vi "CDF Mechanism Controller.vi"(8 "error in":errorcluster) -> ()   [LabVIEW 2015]
doc: "This VI executes continuously carrying out the current operation and responding to updates or new operations. It will often contain the timing or control code that is difficult to place directly in TeleOp. This VI generally opens all sensors and motors and isolates the rest of the robot code from knowing how the operations are carried out."
uses:
  CDF Mechanism Setpoints.ctl
  CDF Mechanism Operations.ctl
  <vilib>/Rock Robotics/WPI/CAN/TalonSRX/WPI_CANTalonSRX_APIControlMode.ctl
  <vilib>/Rock Robotics/WPI/CAN/TalonSRX/WPI_CANTalonSRX_BrakeOverride.ctl
  <vilib>/Rock Robotics/WPI/CAN/TalonSRX/WPI_CANTalonSRX_APIFeedbackSelect.ctl
  Support Code/OnButton/OnButtonSingle.vi
  <vilib>/Rock Robotics/WPI/MotorControl/WPI_MotorControlOpenCANTalonSRX.vi
panel:
  out "Current\nCmd":string
  # "Tip: It may be helpful to observe inputs and sensor values.\nYou may also want to display tuning or debugging controls."
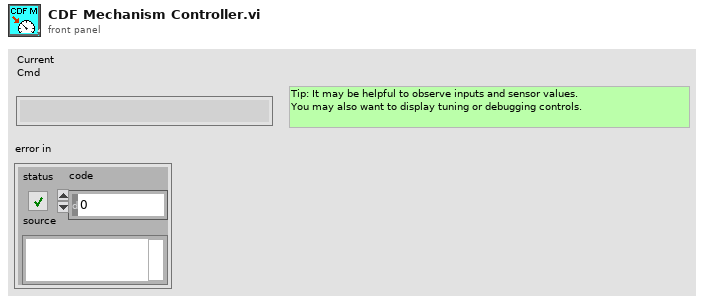
[diagram p1: front panel]
types:
  T1 = typedef "CDF Mechanism Setpoints.ctl" = cluster{"Operation":T2, "Setpoint":dbl, "Duration":dbl, "Setpoint (Top is = True )":bool}
  T2 = typedef "CDF Mechanism Operations.ctl" = enum16{"Reserve", "Read Current", "Immediate", "Idle", "Flip", "Set", "Manual"}
  T3 = typedef "Command Status Info.ctl" = cluster{"Name":string, "Status":T4, "notifier out":T5}
  T4 = typedef "Completion Status.ctl" = enum16{"Successful", "Aborted", "Incomplete"}
  T5 = typedef "Completion Notifier.ctl" = refnum<notifier>
  T6 = cluster{"Default Command":T1, "Command Timing":cluster{"Start Time (ms)":u32, "Iterations":i32}, "Command Arguments":cluster{"Command Info":T3, "Description":string, "Default Command":T1, "notifier out":refnum<notifier>, "Subsystem Name":string}}
  T7 = typedef "WPI_CANTalonSRX_APIFeedbackSelect.ctl" = enum16{"Digital Quadrature Encoder", "Analog Potentiometer", "Analog Encoder", "Count on Quad-A (Rising-Edge)", "Count on Quad-A (Falling-Edge)", "CTR Magnetic Enc (Absolute)", "CTR Magnetic Enc (Relative)", "Pulse Width"}
  T8 = typedef "WPI_CANTalonSRX_BrakeOverride.ctl" = enum8{"No Override", "Override to Coast", "Override to Brake"}
  T9 = typedef "WPI_CANTalonSRX_APIControlMode.ctl" = enum8{"Percent VBus", "Speed", "Position", "Slave", "Unchanged / Invalid", "Voltage Compensation", "Current", "Motion Profile"}
  T10 = typedef "WPI_MotorControlDeviceRef.ctl" = cluster{"DeviceStatus":errorcluster, "Type":T11, "PWM":cluster{"PWM Channel":T12, "DeadBand":T13}, "CAN":cluster{"Device Number":u8, "Control Mode":T14, "Semaphore":T15, "Max Vout":dbl, "TalonSRX Control Mode":T9}, "Invert":bool}
  T11 = typedef "WPI_MotorControlType.ctl" = enum16{"PWM", "CAN", "CANTalonSRX"}
  T12 = typedef "FPGA_DIOPWMChannel.ctl" = enum8{"PWM 0", "PWM 1", "PWM 2", "PWM 3", "PWM 4", "PWM 5", "PWM 6", "PWM 7", "PWM 8", "PWM 9", "PWM MXP 0", "PWM MXP 1", "PWM MXP 2", "PWM MXP 3", "PWM MXP 4", "PWM MXP 5", "PWM MXP 6", "PWM MXP 7", "PWM MXP 8", "PWM MXP 9", "Invalid"}
  T13 = typedef "WPI_PWMDeadband.ctl" = cluster{"Name":string, "maxPositivePwm":i32, "minPositivePwm":i32, "centerPwm":i32, "maxNegativePwm":i32, "minNegativePwm":i32, "angularRange":u16}
  T14 = typedef "WPI_CANJaguar_ControlMode.ctl" = enum8{"Percent VBus", "Current", "Speed", "Position", "Voltage"}
  T15 = typedef "Semaphore RefNum" = refnum<k1>
  T16 = typedef "WPI_CANTalonSRX_GlobalStatus.ctl" = cluster{"Applied Throttle":dbl, "Module Enabled":bool, "CAN Error":errorcluster, "Closed Loop Error":dbl, "Forward Limit Switch Closed":bool, "Reverse Limit Switch Closed":bool, "Sensor Position":dbl, "Sensor Velocity":dbl, "Current":dbl, "Sticky Fault - Over Temp":bool, "Sticky Fault - Under Voltage":bool, "Sticky Fault - Forward Limit":bool, "Sticky Fault - Reverse Limit":bool, "Sticky Fault - Forward Soft Limit":bool, "Sticky Fault - Reverse Soft Limit":bool, "Brake is Enabled":bool, "Encoder Position":dbl, "Encoder Velocity":dbl, "Encoder Index Count":dbl, "Encoder A Pin State":bool, "Encoder B Pin State":bool, "Encoder Index Pin State":bool, "Analog In":dbl, "Analog In Velocity":dbl, "Temperature (C)":dbl, "Battery Voltage":dbl, "Control 5 Is Supported":bool, "Current Profile Slot Select":dbl, "Pos Div 8":bool, "Vel Div 4":bool, "Pulse Width Position":i32, "Pulse Width Velocity":i32, "Pulse Width Rise To Rise (us)":i32, "Pulse Width Rise To Fall (us)":i32, "Mot Prof Active Is Under Run":bool, "Mot Prof Active Has Under Run":bool, "Mot Prof Active Is Last":bool, "Mot Prof Active Velocity Only":bool, "Mot Prof Active Is Valid":bool, "Mot Prof Buffer Is Full":bool, "Mot Prof Active Profile Slot Select":i32, "Mot Prof NextID":i32, "Mot Prof Count":i32, "Mot Prof Active Velocity":dbl, "Mot Prof Active Position":dbl, "Mot Prof Output Enable":i32}
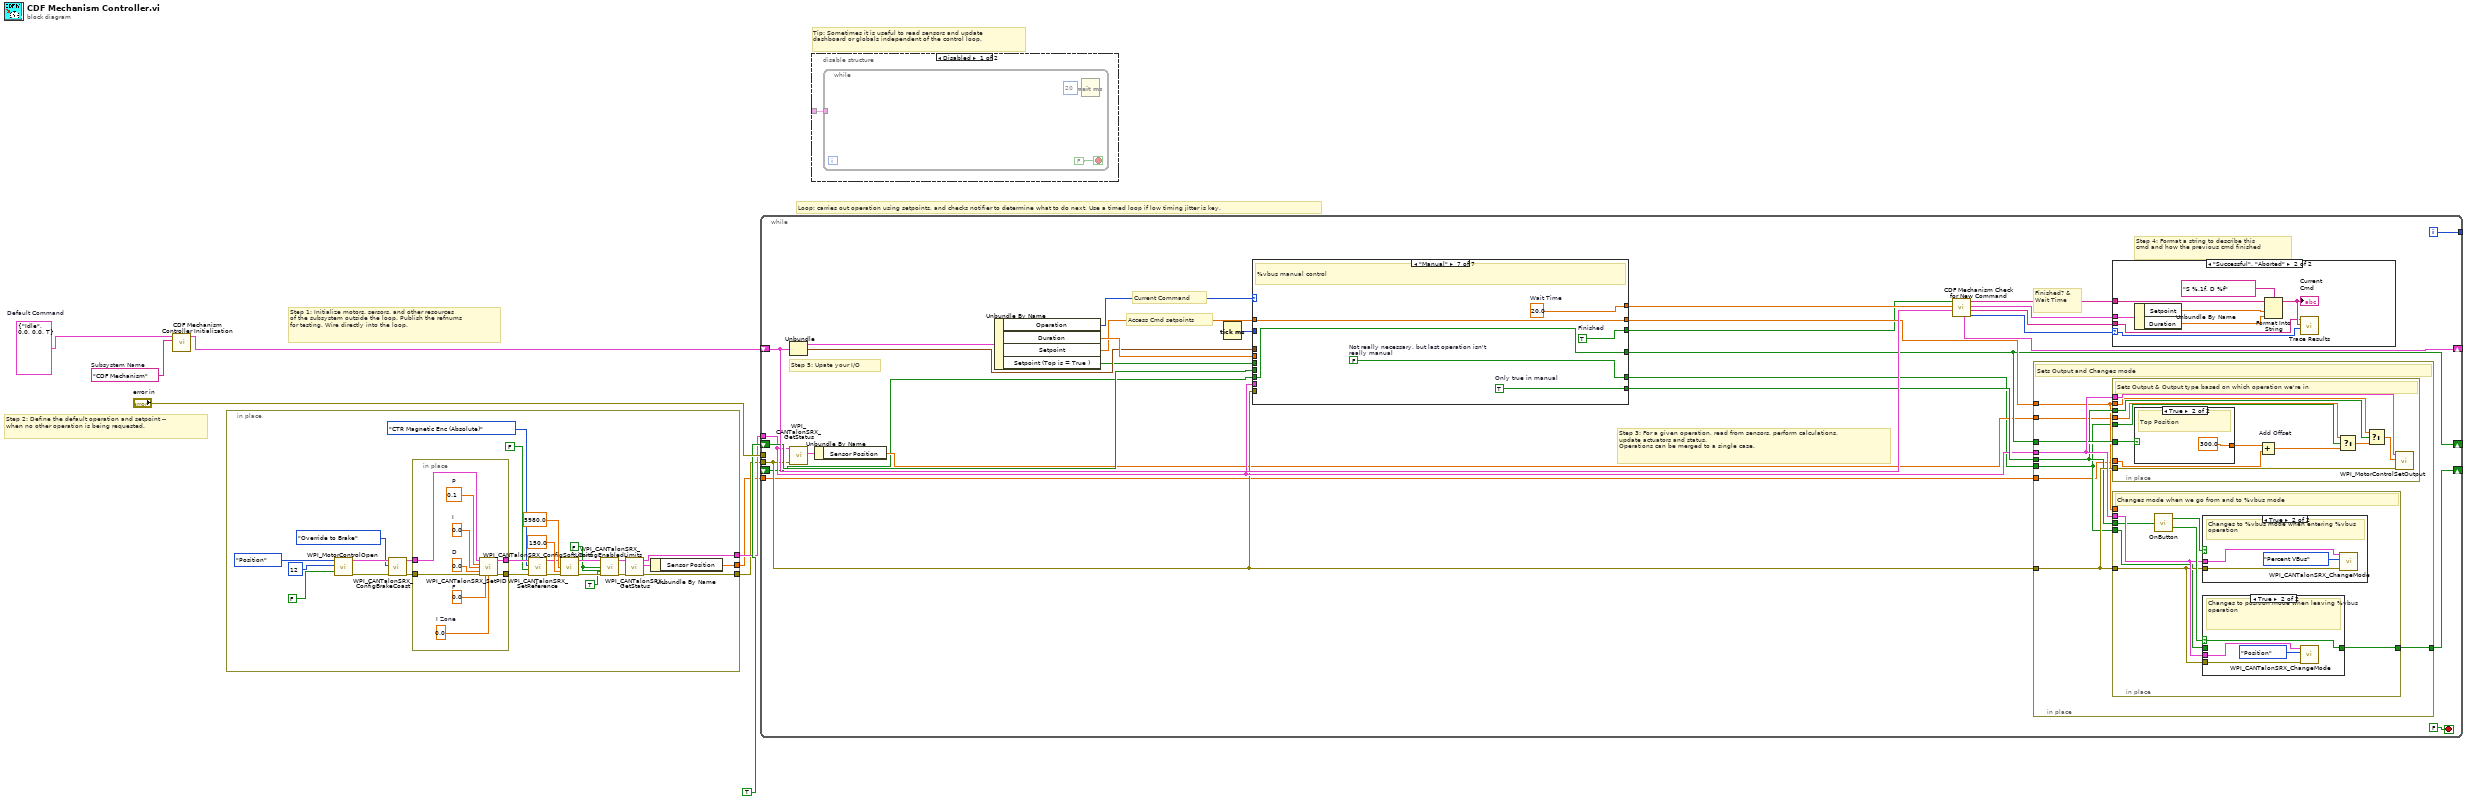
[diagram p0: block diagram]
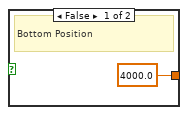
[diagram p3: hidden frame]
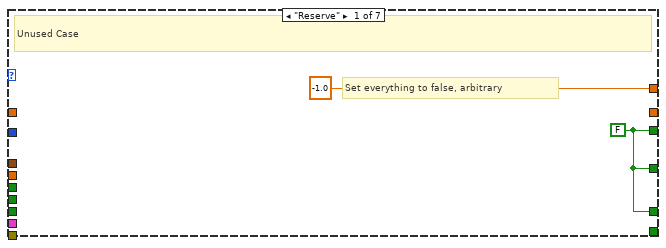
[diagram p7: hidden frame]
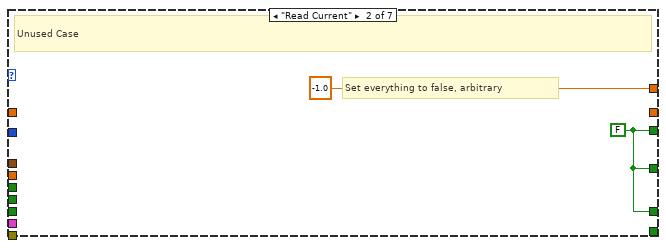
[diagram p8: hidden frame]
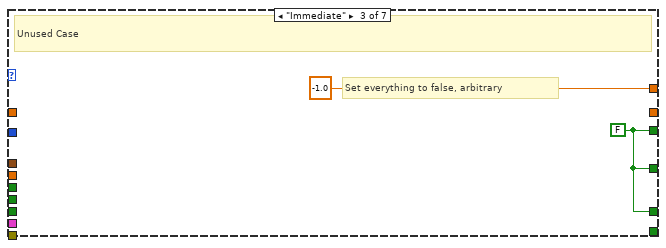
[diagram p9: hidden frame]
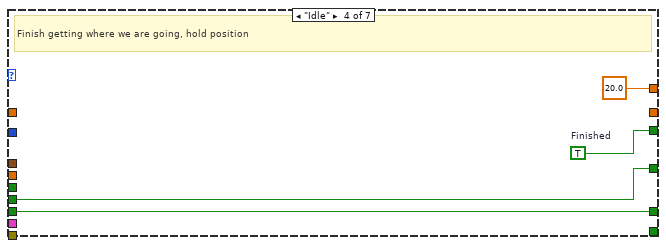
[diagram p10: hidden frame]
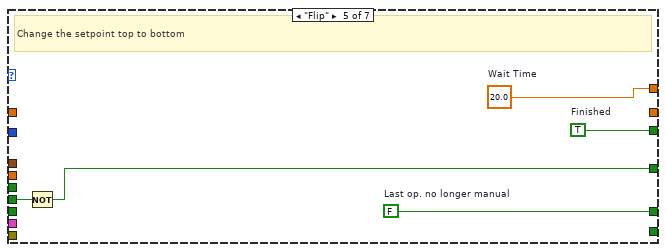
[diagram p11: hidden frame]
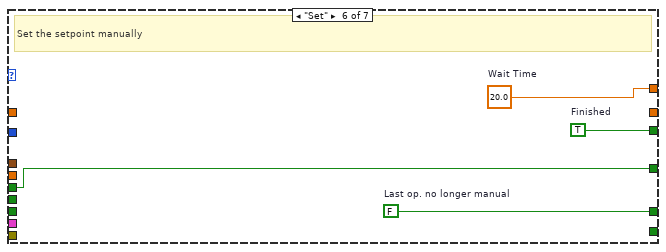
[diagram p12: hidden frame]
diagram:
  w5 = T1 {"Operation"=enum."Idle", "Setpoint"=0.0, "Duration"=0.0, "Setpoint (Top is = True )"=TRUE}  # Default Command
  w6 = "CDF Mechanism"  # Subsystem Name
  # "Tip: Sometimes it is useful to read sensors and update\ndashboard or globals independent of the control loop."
  # "Step 2: Define the default operation and setpoint --\nwhen no other operation is being requested."
  # "Step 1: Initialize motors, sersors, and other resources\nof the subsystem outside the loop. Publish the refnums\nfor testing. Wire directly into the loop."
  # "Loop: carries out operation using setpoints, and checks notifier to determine what to do next. Use a timed loop if low timing jitter is key."
  n1 = call "CDF Mechanism Controller Initialization.vi"("Subsystem Name"=w6, "Default Command"=w5) -> ("Command Info"=w7:T6)  [unwired: 9 in]
  n2 = in-place {
    in-place-border: [w13] -> w3
    in-place-border: [w11] -> w2
    in-place-border: [w9] -> w1
    w20 = FALSE ("Forward Limit Switch Enable")
    w21 = TRUE ("Reverse Soft Limit Enable")
    n3 = call-poly <vilib>:"WPI_MotorControlOpen.vi"("Invert"=FALSE, "Device Number"=u8 12, "Control Mode"=WPI_CANTalonSRX_APIControlMode."Position") -> ("error out"=w30:errorcluster, "MotorControlDeviceRef"=w29:T10)  [unwired: 7 in]
    n4 = call <vilib>:"WPI_CANTalonSRX_ConfigBrakeCoast.vi"("error in (no error)"=w30, "Brake / Coast Mode"=WPI_CANTalonSRX_BrakeOverride."Override to Brake", "CAN Talon SRX Ref"=w29) -> ("error out"=w32:errorcluster, "CAN Talon SRX Ref"=w31:T10)  [unwired: 7 in]
    n5 = in-place {
      in-place-border: w32 -> [w43]
      in-place-border: w31 -> [w42]
      in-place-border: [w41] -> w18
      in-place-border: [w40] -> w17
      w35 = 0.0  # I Zone
      w36 = 0.0  # F
      w37 = 0.0  # D
      w38 = 0.0  # I
      w39 = 0.1  # P
      n6 = call <vilib>:"WPI_CANTalonSRX_SetPID.vi"("CAN Talon SRX Ref"=w42, "P"=w39, "I"=w38, "D"=w37, "error in (no error)"=w43, "F"=w36, "I Zone"=w35) -> ("CAN Talon SRX Ref"=w41:T10, "error out"=w40:errorcluster)  [unwired: 7 in]
    }
    n7 = call <vilib>:"WPI_CANTalonSRX_SetReference.vi"("error in (no error)"=w17, "Reverse Feedback Sensor"=FALSE, "Feedback Reference"=WPI_CANTalonSRX_APIFeedbackSelect."CTR Magnetic Enc (Absolute)", "CAN Talon SRX Ref"=w18) -> ("error out"=w16:errorcluster, "CAN Talon SRX Ref"=w19:T10)  [unwired: 6 in]
    n8 = call <vilib>:"WPI_CANTalonSRX_ConfigSoftLimits.vi"("CAN Talon SRX Ref"=w19, "Forward Limit Position"=5980.0, "Reverse Limit Position"=150.0, "error in (no error)"=w16) -> ("CAN Talon SRX Ref"=w24:T10, "error out"=w22:errorcluster)  [unwired: 10 in]
    n9 = call <vilib>:"WPI_CANTalonSRX_ConfigEnabledLimits.vi"("CAN Talon SRX Ref"=w24, "Forward Limit Switch Enable"=w20, "Reverse Limit Switch Enable"=w20, "error in (no error)"=w22, "Forward Soft Limit Enable"=w21, "Reverse Soft Limit Enable"=w21) -> ("CAN Talon SRX Ref"=w23:T10, "error out"=w12:errorcluster)  [unwired: 8 in]
    n10 = call <vilib>:"WPI_CANTalonSRX_GetStatus.vi"("error in (no error)"=w12, "CAN Talon SRX Ref"=w23) -> ("error out"=w11:errorcluster, "Talon SRX Status"=w10:T16, "CAN Talon SRX Ref"=w13:T10)  [unwired: 7 in]
    n11 = Unbundle By Name(w10) -> ("Sensor Position"=w9:dbl)
  }
  n12 = while {
    shift-right: [w63] -> _
    shift-left: w7 -> [w64]
    tunnel: [w71] -> _
    tunnel: "error in" -> [_]
    shift-right: [w54] -> _
    shift-left: TRUE -> [w57]
    tunnel: w3 -> [w52]
    tunnel: w2 -> [w51]
    shift-right: [w48] -> _
    shift-left: _ -> [w46]
    tunnel: w1 -> [w44]
    i -> [w71]
    stop <- FALSE stop-if-true
    # "Step 5: Upate your I/O"
    # "Step 4: Format a string to describe this\ncmd and how the previous cmd finished"
    # "Current Command"
    # "Access Cmd setpoints"
    # "Finished? &\nWait Time"
    # "Step 3: For a given operation, read from sensors, perform calculations,\nupdate actuators and status.\nOperations can be merged to a single case."
    n13 = Unbundle(w64) -> ("Default Command"=w70:T1, "Command Timing"=w66:cluster{"Start Time (ms)":u32, "Iterations":i32})  [unwired: 1 out]
    n14 = call <vilib>:"WPI_CANTalonSRX_GetStatus.vi"("error in (no error)"=w51, "CAN Talon SRX Ref"=w52) -> ("Talon SRX Status"=w50:T16)  [unwired: 7 in, 2 out]
    n15 = Unbundle By Name(w50) -> ("Sensor Position"=w49:dbl)
    n16 = Unbundle By Name(w70) -> ("Operation"=w69:T2, "Duration"=w68:dbl, "Setpoint"=w65:dbl, "Setpoint (Top is = True )"=w56:bool)
    n17 = Tick Count (ms)() -> (millisecond timer value=w67:u32)
    n18 = case shown="\"Manual\"" w69 {
      tunnel: [-1.0 -1.0 -1.0 20.0 w130 w136 w139] -> w62
      tunnel: [w119 w121 w123 w127 w131 w134 w140] -> w45
      tunnel: w66 -> [_ _ _ _ _ _ _]
      tunnel: w68 -> [_ _ _ _ _ _ _]
      tunnel: w67 -> [_ _ _ _ _ _ _]
      tunnel: w65 -> [_ _ _ _ _ _ w142]
      tunnel: w57 -> [_ _ _ w128 w133 _ _]
      tunnel: [w119 w121 w123 w128 w132 w137 w138] -> w54
      tunnel: w56 -> [_ _ _ _ _ w137 _]
      tunnel: w52 -> [_ _ _ _ _ _ _]
      tunnel: w51 -> [_ _ _ _ _ _ _]
      tunnel: [_ _ _ _ _ _ w143] -> w53
      tunnel: [_ _ _ _ _ _ w142] -> w55
      tunnel: [w119 w121 w123 w125 w129 w135 w141] -> w47
      tunnel: w46 -> [_ _ _ w125 _ _ w138]
      frame "Reserve" {
        w119 = FALSE ("ignore previous (F)")
        # "Set everything to false, arbitrary"
        # "Unused Case"
      }
      frame "Read Current" {
        w121 = FALSE ("ignore previous (F)")
        # "Set everything to false, arbitrary"
        # "Unused Case"
      }
      frame "Immediate" {
        w123 = FALSE ("ignore previous (F)")
        # "Set everything to false, arbitrary"
        # "Unused Case"
      }
      frame "Idle" {
        w127 = TRUE  # Finished
        # "Finish getting where we are going, hold position"
      }
      frame "Flip" {
        w129 = FALSE  # Last op. no longer manual
        w130 = 20.0  # Wait Time
        w131 = TRUE  # Finished
        # "Change the setpoint top to bottom"
        n19 = Not(x=w133) -> (.not. x?=w132:bool)
      }
      frame "Set" {
        w134 = TRUE  # Finished
        w135 = FALSE  # Last op. no longer manual
        w136 = 20.0  # Wait Time
        # "Set the setpoint manually"
      }
      frame "Manual" {
        w139 = 20.0  # Wait Time
        w140 = TRUE  # Finished
        w141 = FALSE  # Not really necessary, but last operation isn't really manual
        w143 = TRUE  # Only true in manual
        # "%vbus manual control"
      }
    }
    n20 = call "CDF Mechanism Check for New Command.vi"("Current Command"=w64, "Wait time (ms)"=w62, "Finished?"=w45) -> ("Completion"=w58:T4, "Subsystem Name"=w59:string, "Current Command"=w60:T1, "Initial Trace String"=w61:string, "NextCommand"=w63:T6)  [unwired: 4 in]
    n21 = in-place {
      in-place-border: w55 -> [w77]
      in-place-border: w52 -> [w81]
      in-place-border: w51 -> [w80]
      in-place-border: w54 -> [w79]
      in-place-border: w53 -> [w78]
      in-place-border: w47 -> [w74]
      in-place-border: w49 -> [w76]
      in-place-border: [w75] -> w48
      in-place-border: w44 -> [w73]
      # "Sets Output and Changes mode"
      n22 = in-place {
        in-place-border: w81 -> [w93]
        in-place-border: w80 -> [w92]
        in-place-border: w79 -> [w91]
        in-place-border: w78 -> [w88]
        in-place-border: w77 -> [w90]
        in-place-border: w74 -> [w86]
        in-place-border: w76 -> [w85]
        in-place-border: w73 -> [w82]
        # "Sets Output & Output type based on which operation we're in"
        n23 = case shown="True" w91 {
          tunnel: [4000.0 300.0] -> w84
          frame False {
            # "Bottom Position"
          }
          frame True {
            # "Top Position"
          }
        }
        n24 = Add "Add Offset"(x=w84, y=w82) -> (x+y=w83:dbl)
        n25 = Select(t=w85, s=w86, f=w83) -> (s? t:f=w87:dbl)
        n26 = Select(t=w90, s=w88, f=w87) -> (s? t:f=w89:dbl)
        n27 = call <vilib>:"WPI_MotorControlSetOutput.vi"("error in (no error)"=w92, "Output"=w89, "MotorControlDevRef"=w93) -> ()  [unwired: 6 in, 3 out]
      }
      n28 = in-place {
        in-place-border: w77 -> [_]
        in-place-border: w81 -> [w101]
        in-place-border: w80 -> [w99]
        in-place-border: w78 -> [w98]
        in-place-border: [w97] -> w75
        in-place-border: w74 -> [w96]
        # "Changes mode when we go from and to %vbus mode"
        n29 = call-poly "OnButton.vi"("Input"=w98) -> ("Pressed"=w100:bool, "Released"=w102:bool)
        n30 = case shown="True" w100 {
          tunnel: w99 -> [_ w109]
          tunnel: w101 -> [_ w108]
          frame False {
          }
          frame True {
            # "Changes to %vbus mode when entering %vbus operation"
            n31 = call <vilib>:"WPI_CANTalonSRX_ChangeMode.vi"("error in (no error)"=w109, "Control Mode"=WPI_CANTalonSRX_APIControlMode."Percent VBus", "CAN Talon SRX Ref"=w108) -> ()  [unwired: 7 in, 2 out]
          }
        }
        n32 = case shown="True" w102 {
          selector: w102 -> [_ w104]
          tunnel: w101 -> [_ w106]
          tunnel: w99 -> [_ w105]
          tunnel: [w103 w104] -> w97
          tunnel: w96 -> [w103 _]
          frame False {
          }
          frame True {
            # "Changes to position mode when leaving %vbus operation"
            n33 = call <vilib>:"WPI_CANTalonSRX_ChangeMode.vi"("error in (no error)"=w105, "Control Mode"=WPI_CANTalonSRX_APIControlMode."Position", "CAN Talon SRX Ref"=w106) -> ()  [unwired: 7 in, 2 out]
          }
        }
      }
    }
    n34 = case shown="\"Successful\", \"Aborted\"" w58 {
      selector: w58 -> [_ w118]
      tunnel: w61 -> [_ w114]
      tunnel: w60 -> [_ w115]
      tunnel: w59 -> [_ w111]
      frame "Incomplete", Default {
        # "Continuing current command"
      }
      frame "Successful", "Aborted" {
        # "Report and setup for next command"
        n35 = Unbundle By Name(w115) -> ("Setpoint"=w117:dbl, "Duration"=w112:dbl)
        n36 = Format Into String(format string="S %.1f, D %f", initial string=w114, w117, w112) -> (resulting string=w113:string)  [unwired: 1 in, 1 out]
        "Current\nCmd" <- w113
        n37 = call <vilib>:"Trace Results.vi"("Status of previous command"=w118, "Description"=w113, "Subsystem"=w111) -> ()  [unwired: 9 in]
      }
    }
  }
  n38 = disable-structure shown="Disabled" {
    disable-tunnel: _ -> [w144 _]
    frame Disabled {
      n39 = while {
        tunnel: w144 -> [_]
        stop <- FALSE stop-if-true
        n40 = Wait (ms)(milliseconds to wait=u32 20) -> ()  [unwired: 1 out]
      }
    }
    frame Enabled {
    }
  }
